vi "2.-WaveformGraph_WaveformChart.vi"() -> ()   [LabVIEW 2020]
panel:
  in  "Tab Control":enum32{"Page 4", "Page 1", "Page 2", "Page 3"}(tab)
  out "Waveform Graph 4":dbl[][](graph)
  out "Waveform Graph 2":cluster{dbl, dbl, dbl[]}(graph)
  out "Waveform Chart 2":T1(graph)
  out "Waveform Chart":dbl(graph)
  out "Waveform Graph":cluster{dbl, dbl, dbl[]}(graph)
  out "Waveform Graph 3":dbl[](graph)
  in  "stop":bool
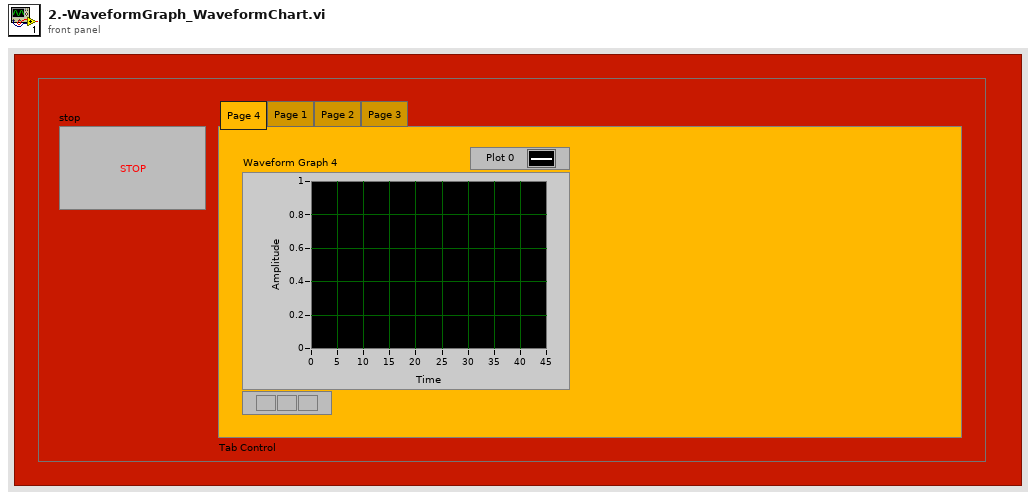
[diagram p1: front panel]
types:
  T1 = cluster{"number: 0 to 1":dbl, "number: 0 to 1":dbl, "number: 0 to 1":dbl}
  T2 = cluster{"number: 0 to 1":dbl, "number: 0 to 1":dbl, "number: 0 to 1":dbl}[]
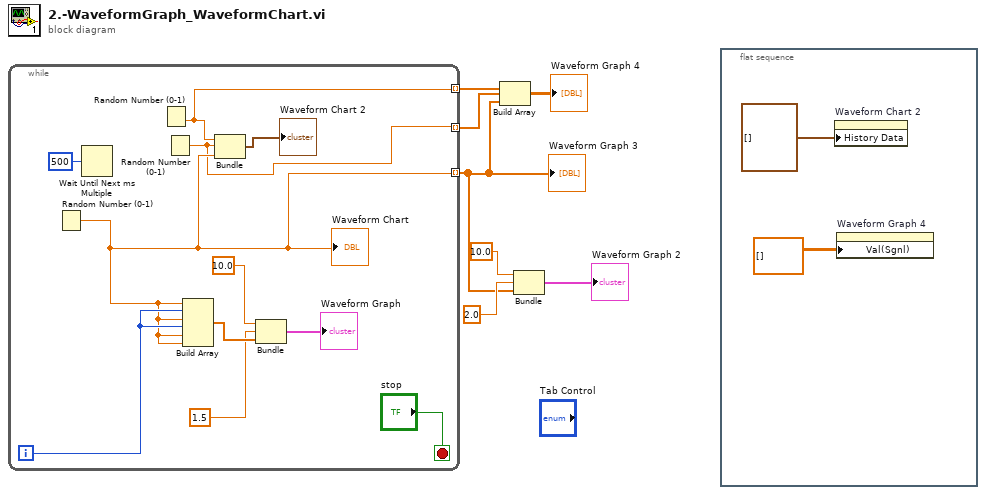
[diagram p0: block diagram]
diagram:
  n1 = while {
    tunnel: [w11] -> w2 mode=indexing
    tunnel: [w9] -> w4 mode=indexing
    tunnel: [w8] -> w3 mode=indexing
    i -> [w12]
    stop <- "stop" stop-if-true
    n2 = Random Number (0-1)() -> (number: 0 to 1=w11:dbl)
    "Waveform Chart" <- w11
    n3 = Wait Until Next ms Multiple(millisecond multiple=u32 500) -> ()  [unwired: 1 out]
    n4 = Random Number (0-1)() -> (number: 0 to 1=w9:dbl)
    n5 = Random Number (0-1)() -> (number: 0 to 1=w8:dbl)
    n6 = Build Array(w11, w12, w11, w12, w11, w11) -> (w16:dbl[])
    n7 = Bundle("number: 0 to 1"=w9, "number: 0 to 1"=w8, "number: 0 to 1"=w11) -> (→"Waveform Chart 2":T1)  [unwired: 1 in]
    n8 = Bundle(10.0, 1.5, w16) -> (→"Waveform Graph":cluster{dbl, dbl, dbl[]})  [unwired: 1 in]
  }
  "Waveform Graph 3" <- w2
  n9 = Build Array(w4, w3, w2) -> (→"Waveform Graph 4":dbl[][])
  n10 = Bundle(10.0, 2.0, w2) -> (→"Waveform Graph 2":cluster{dbl, dbl, dbl[]})  [unwired: 1 in]
  n11 = flat-sequence {
    frame #0 {
      n12 = property on="Waveform Chart 2" class="WaveformChart (strict)"("History Data"=T2 []) -> ()  [unwired: 2 in, 2 out]
      n13 = property on="Waveform Graph 4" class="WaveformGraph (strict)"("Val(Sgnl)"=dbl[][] [] ("Value (Signaling)")) -> ()  [unwired: 2 in, 2 out]
    }
  }
